vi "Import - Buffered Tx Packet.vi"(7 "Tx Packet":T1 {"threadOptions"."pclDecimation" max=16 step=1; "threadOptions"."loopPeriod" max=16 step=1; "threadOptions"."targetPriority" min=-2 max=16 step=1; "threadOptions"."targetProcessor" min=-2 max=16 step=1; "Endianness" items=["big-endian"=0, "little-endian"=2]}, 8 "error in (no error)":errorcluster, 11 "Device Item Ref in":T13 format="%.0x") -> (0 "error out":errorcluster)   [LabVIEW 2016, in "UDP-Custom-Device System Explorer.lvlib"]
uses:
  UDP-Custom-Device System Explorer.lvlib
  <vilib>/NI Veristand/Custom Device API/Custom Device Item Ref.ctl
  Types/XML - New/ImpExp - Tx Packet Data.ctl
  <vilib>/NI Veristand/Custom Device API/Custom Device Item Info.ctl
  Shared/Types/Shared - Channel Data Type.ctl
  Shared/Types/Shared - Buffered.PacketInfo.ctl
  Shared/Types/Shared - Pointer Encoding.ctl
  Shared/Types/Shared - Receive Buffer Options.ctl
  Shared/Types/Shared - Transmit Buffer Options.ctl
  Shared/Types/Shared - Transmit Flag Options.ctl
  Shared/Types/Shared - Transmit Echo Options.ctl
  Types/Threading/Thread Configuration.ctl
  Types/Threading/Thread Sync Reference.ctl
  Shared/Types/Shared - Thread Management.ctl
  Property Accessors/Shared Packet Accessors.lvlib
  Property Accessors/Tx Packet Accessors.lvlib
  <vilib>/NI VeriStand/Custom Device API/Custom Device API.lvlib
  <vilib>/NI VeriStand/Custom Device Tools/Custom Device Utility Library/Custom Device Utility Library.lvlib
  Property Accessors/Buffered Data Packet.lvlib
  Shared/UDP-Custom-Device Shared.lvlib
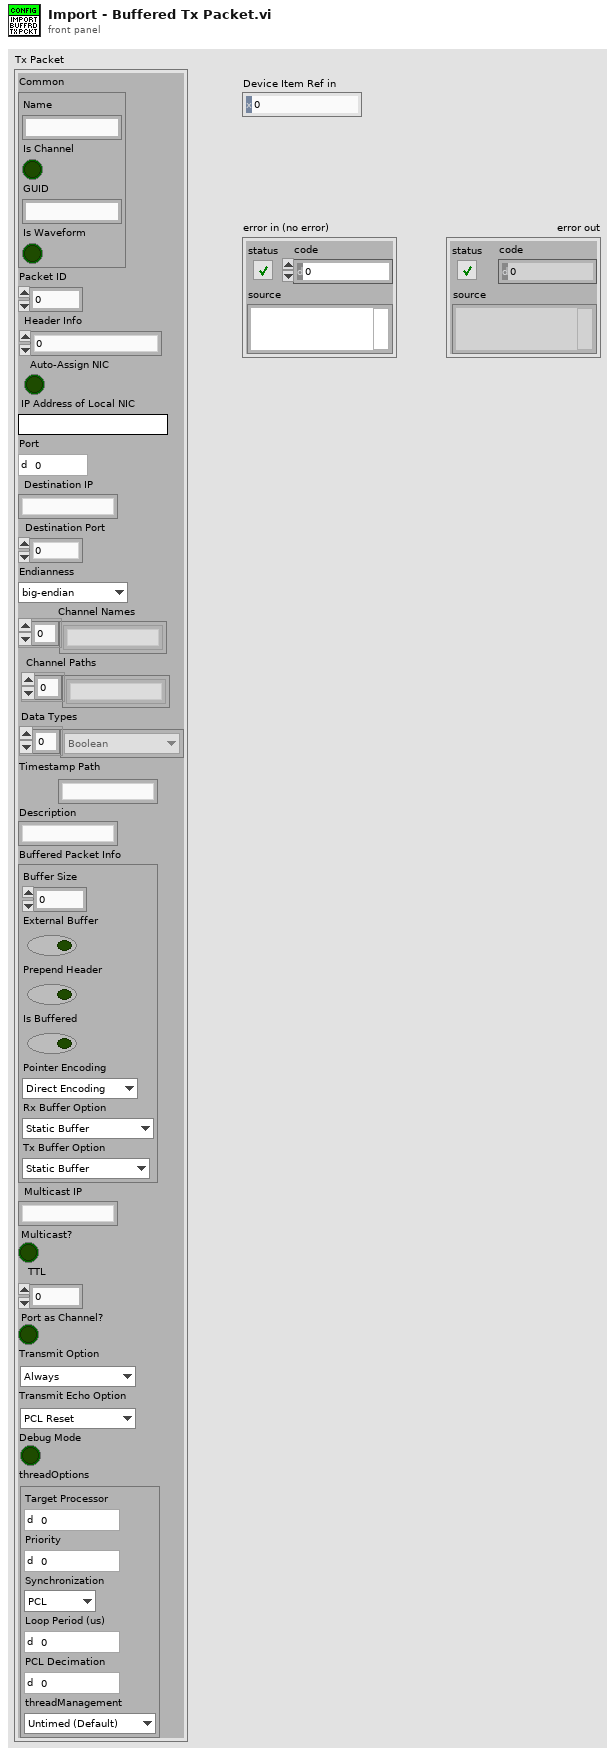
[diagram p1: front panel]
types:
  T1 = typedef "UDP-Custom-Device System Explorer.lvlib/ImpExp - Tx Packet Data.ctl" = cluster{"Common":T2, "Packet ID":i32, "Header Info":u32, "Auto-Assign NIC":bool, "IP Address of Local NIC":string, "Port":u16, "Destination IP":string, "Destination Port":u16, "Endianness":u16, "Channel Names":string[], "Channel Paths":string[], "Data Types":T3[], "Timestamp Path":string, "Description":string, "Buffered Packet Info":T4, "Multicast IP":string, "Multicast?":bool, "TTL":u16, "Port as Channel?":bool, "Transmit Option":T8, "Transmit Echo Option":T9, "Debug Mode":bool, "threadOptions":T10}
  T2 = typedef "Custom Device API.lvlib/Custom Device Item Info.ctl" = cluster{"Name":string, "Is Channel":bool, "GUID":string, "Is Waveform":bool}
  T3 = typedef "UDP-Custom-Device Shared.lvlib/Shared - Channel Data Type.ctl" = enum16{"Boolean", "Single", "Double", "I8", "I16", "I32", "I64", "U8", "U16", "U32", "U64"}
  T4 = typedef "UDP-Custom-Device Shared.lvlib/Shared - Buffered.PacketInfo.ctl" = cluster{"Buffer Size":i32, "External Buffer":bool, "Prepend Header":bool, "Is Buffered":bool, "Pointer Encoding":T5, "Rx Buffer Option":T6, "Tx Buffer Option":T7}
  T5 = typedef "UDP-Custom-Device Shared.lvlib/Shared - Pointer Encoding.ctl" = enum16{"Direct Encoding", "Conversion Encoding"}
  T6 = typedef "UDP-Custom-Device Shared.lvlib/Shared - Receive Buffer Options.ctl" = enum16{"Static Buffer", "Circular Buffer", "Circular Buffer + Size", "Internal Cache", "Internal Cache + Size"}
  T7 = typedef "UDP-Custom-Device Shared.lvlib/Shared - Transmit Buffer Options.ctl" = enum16{"Static Buffer", "FIFO Buffer", "FIFO Buffer + Port"}
  T8 = typedef "UDP-Custom-Device Shared.lvlib/Shared - Transmit Flag Options.ctl" = enum16{"Always", "One-Shot", "Toggle"}
  T9 = typedef "UDP-Custom-Device Shared.lvlib/Shared - Transmit Echo Options.ctl" = enum16{"PCL Reset", "Counter", "Mirror"}
  T10 = typedef "UDP-Custom-Device System Explorer.lvlib/Thread Configuration.ctl" = cluster{"targetProcessor":i8, "targetPriority":i16, "Synchronization":T11, "loopPeriod":u32, "pclDecimation":u16, "threadManagement":T12}
  T11 = typedef "UDP-Custom-Device System Explorer.lvlib/Thread Sync Reference.ctl" = enum16{"PCL", "Async"}
  T12 = typedef "UDP-Custom-Device Shared.lvlib/Shared - Thread Management.ctl" = enum16{"Untimed (Default)", "Timed (High Priority)"}
  T13 = typedef "Custom Device API.lvlib/Custom Device Item Ref.ctl" = u64
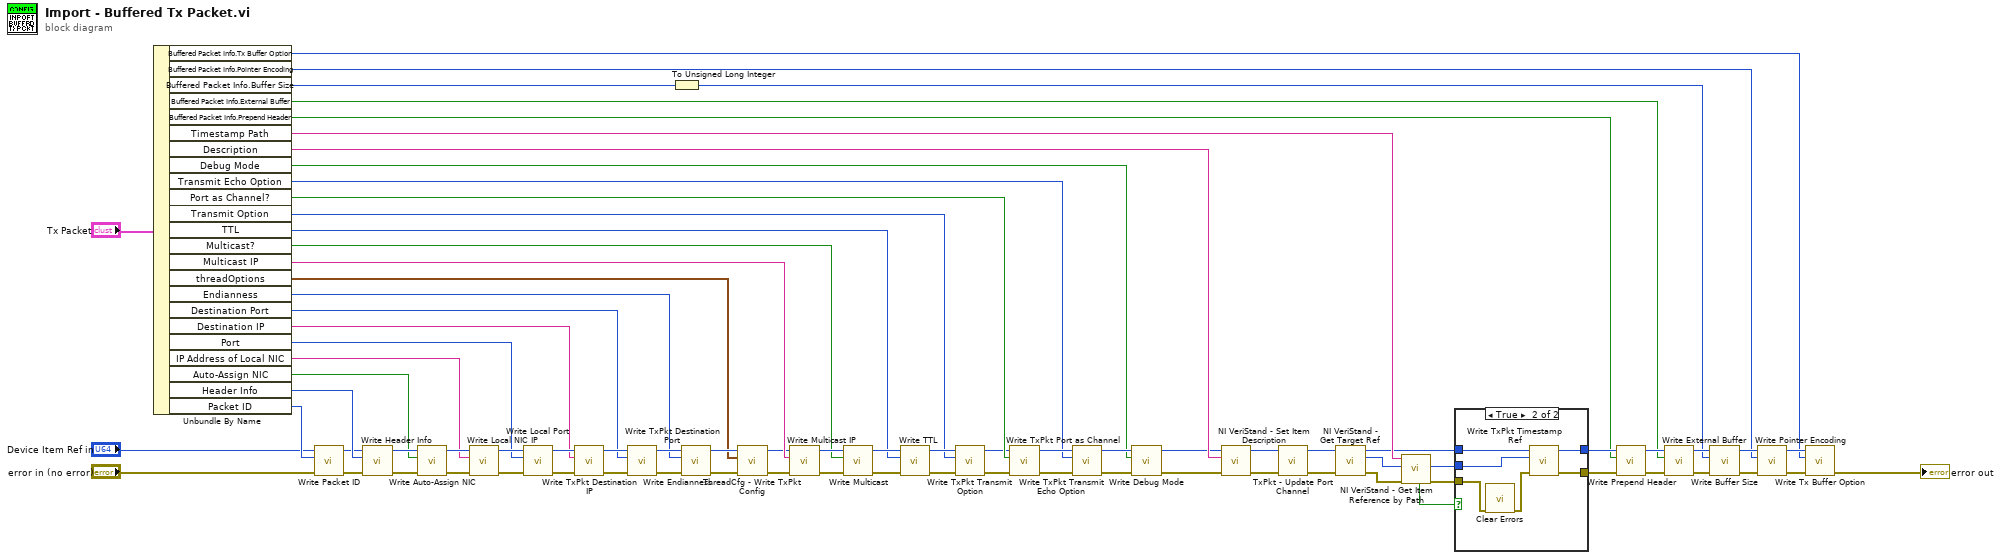
[diagram p0: block diagram]
diagram:
  n1 = Unbundle By Name("Tx Packet") -> ("Buffered Packet Info.Tx Buffer Option"=w14:T7, "Buffered Packet Info.Pointer Encoding"=w28:T5, "Buffered Packet Info.Buffer Size"=w39:i32, "Buffered Packet Info.External Buffer"=w40:bool, "Buffered Packet Info.Prepend Header"=w41:bool, "Timestamp Path"=w51:string, "Description"=w57:string, "Debug Mode"=w6:bool, "Transmit Echo Option"=w11:T9, "Port as Channel?"=w27:bool, "Transmit Option"=w22:T8, "TTL"=w31:u16, "Multicast?"=w32:bool, "Multicast IP"=w33:string, "threadOptions"=w4:T10, "Endianness"=w58:u16, "Destination Port"=w61:u16, "Destination IP"=w62:string, "Port"=w63:u16, "IP Address of Local NIC"=w64:string, "Auto-Assign NIC"=w73:bool, "Header Info"=w78:u32, "Packet ID"=w79:i32)
  n2 = call "Write Packet ID.vi"("error in (no error)"="error in (no error)", "Packet ID"=w79, "Node Ptr"="Device Item Ref in") -> ("error out"=w76:errorcluster, "Node Ptr out"=w77:T13)  [unwired: 7 in]
  n3 = call "Write Header Info.vi"("error in (no error)"=w76, "Header Info"=w78, "Node Ptr"=w77) -> ("error out"=w74:errorcluster, "Node Ptr out"=w75:T13)  [unwired: 7 in]
  n4 = call "Write Auto-Assign NIC.vi"("error in (no error)"=w74, "Auto-Assign NIC"=w73, "Node Ptr"=w75) -> ("error out"=w68:errorcluster, "Node Ptr out"=w72:T13)  [unwired: 7 in]
  n5 = call "Write Local NIC IP.vi"("error in (no error)"=w68, "IP Address of Local NIC"=w64, "Node Ptr"=w72) -> ("error out"=w67:errorcluster, "Node Ptr out"=w71:T13)  [unwired: 7 in]
  n6 = call "Write Local Port.vi"("error in (no error)"=w67, "Port"=w63, "Node Ptr"=w71) -> ("error out"=w66:errorcluster, "Node Ptr out"=w70:T13)  [unwired: 7 in]
  n7 = call "Write TxPkt Destination IP.vi"("error in (no error)"=w66, "Destination IP"=w62, "Node Ptr"=w70) -> ("error out"=w65:errorcluster, "Node Ptr out"=w69:T13)  [unwired: 7 in]
  n8 = call "Write TxPkt Destination Port.vi"("error in (no error)"=w65, "Destination Port"=w61, "Node Ptr"=w69) -> ("error out"=w59:errorcluster, "Node Ptr out"=w60:T13)  [unwired: 7 in]
  n9 = To Unsigned Long Integer(number=w39) -> (unsigned 32bit integer=w38:u32)
  n10 = call "Write Endianness.vi"("error in (no error)"=w59, "Endianness"=w58, "Node Ptr"=w60) -> ("error out"=w3:errorcluster, "Node Ptr out"=w5:T13)  [unwired: 7 in]
  n11 = call "ThreadCfg - Write TxPkt Config.vi"("error in (no error)"=w3, "threadOptions"=w4, "Node Ptr In"=w5) -> ("error out"=w1:errorcluster, "Node Ptr Out"=w2:T13)  [unwired: 7 in]
  n12 = call "Write Multicast IP.vi"("error in (no error)"=w1, "Multicast IP Address"=w33, "Node Ptr"=w2) -> ("error out"=w37:errorcluster, "Node Ptr out"=w35:T13)  [unwired: 7 in]
  n13 = call "Write Multicast.vi"("error in (no error)"=w37, "Multicast"=w32, "Node Ptr"=w35) -> ("error out"=w36:errorcluster, "Node Ptr out"=w34:T13)  [unwired: 7 in]
  n14 = call "Write TTL.vi"("error in (no error)"=w36, "TTL"=w31, "Node Ptr"=w34) -> ("error out"=w24:errorcluster, "Node Ptr out"=w26:T13)  [unwired: 7 in]
  n15 = call "Write TxPkt Transmit Option.vi"("error in (no error)"=w24, "Transmit Options"=w22, "Node Ptr"=w26) -> ("error out"=w23:errorcluster, "Node Ptr out"=w25:T13)  [unwired: 7 in]
  n16 = call "Write TxPkt Port as Channel.vi"("error in (no error)"=w23, "Port as Channel"=w27, "Node Ptr"=w25) -> ("error out"=w12:errorcluster, "Node Ptr out"=w13:T13)  [unwired: 7 in]
  n17 = call "Write TxPkt Transmit Echo Option.vi"("error in (no error)"=w12, "Transmit Echo Options"=w11, "Node Ptr"=w13) -> ("error out"=w8:errorcluster, "Node Ptr out"=w10:T13)  [unwired: 7 in]
  n18 = call "Write Debug Mode.vi"("error in (no error)"=w8, "Debug Mode"=w6, "Node Ptr"=w10) -> ("error out"=w7:errorcluster, "Node Ptr out"=w9:T13)  [unwired: 7 in]
  n19 = call <vilib>:"NI VeriStand - Set Item Description.vi"("error in (no error)"=w7, "Description"=w57, "Item Ref in"=w9) -> ("error out"=w19:errorcluster, "Item Ref out"=w21:T13)  [unwired: 6 in, 1 out]
  n20 = call "TxPkt - Update Port Channel.vi"("error in (no error)"=w19, "Packet Ref in"=w21) -> ("error out"=w18:errorcluster, "Packet Ref out"=w20:T13)  [unwired: 8 in]
  n21 = call <vilib>:"NI VeriStand - Get Target Ref.vi"("error in"=w18, "Item Ref in"=w20) -> ("error out"=w53:errorcluster, "Target Ref"=w54:T13, "Item Ref out"=w50:T13)  [unwired: 6 in, 1 out]
  n22 = call <vilib>:"NI VeriStand - Get Item Reference by Path.vi"("error in (no error)"=w53, "Root Ref"=w54, "Item Path in"=w51) -> ("error out"=w52:errorcluster, "Item Ref"=w49:T13, "Found"=w48:bool)  [unwired: 5 in, 1 out]
  n23 = case shown="True" w48 {
    tunnel: w52 -> [w81 w88]
    tunnel: w50 -> [w82 w87]
    tunnel: w49 -> [_ w86]
    tunnel: [w82 w84] -> w46
    tunnel: [w81 w83] -> w47
    frame False {
    }
    frame True {
      n24 = call <vilib>:"Clear Errors.vi"("error in (no error)"=w88) -> ("error out"=w85:errorcluster)  [unwired: 5 in, 1 out]
      n25 = call "Write TxPkt Timestamp Ref.vi"("error in (no error)"=w85, "Dependent Node Ref"=w86, "Node Ptr"=w87) -> ("error out"=w83:errorcluster, "Node Ptr out"=w84:T13)  [unwired: 7 in]
    }
  }
  n26 = call "Write Prepend Header.vi"("error in (no error)"=w47, "Prepend Header"=w41, "Node Ptr"=w46) -> ("error out"=w45:errorcluster, "Node Ptr out"=w44:T13)  [unwired: 7 in]
  n27 = call "Write External Buffer.vi"("error in (no error)"=w45, "External Buffer"=w40, "Node Ptr"=w44) -> ("error out"=w42:errorcluster, "Node Ptr out"=w43:T13)  [unwired: 7 in]
  n28 = call "Write Buffer Size.vi"("error in (no error)"=w42, "Buffer Size"=w38, "Node Ptr"=w43) -> ("error out"=w29:errorcluster, "Node Ptr out"=w30:T13)  [unwired: 7 in]
  n29 = call "Write Pointer Encoding.vi"("error in (no error)"=w29, "Pointer Encoding"=w28, "Node Ptr"=w30) -> ("error out"=w17:errorcluster, "Node Ptr out"=w15:T13)  [unwired: 7 in]
  n30 = call "Write Tx Buffer Option.vi"("error in (no error)"=w17, "Buffer Option"=w14, "Node Ptr"=w15) -> ("error out"=→"error out":errorcluster)  [unwired: 7 in, 1 out]
